vi "Read.vi"(8 "error in (no error)":errorcluster, 9 "timeout (2000 ms)":i32=2000, 10 "bytes to read (100)":i32=100, 11 "TCPConnection in":refnum<class "Connection.lvclass">) -> (0 "error out":errorcluster, 1 "timed out":bool, 2 "Bytes":u8[](array[numeric]) format="%08b", 3 "TCPConnection out":refnum<class "Connection.lvclass">, 4 "connected":bool)   [LabVIEW 2013, in "MQTT_Connection.lvlib" / "Connection.lvclass"]
uses:
  Connection.lvclass
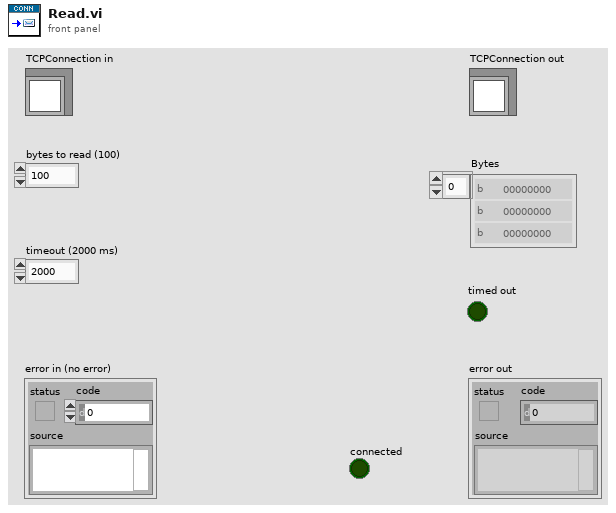
[diagram p1: front panel]
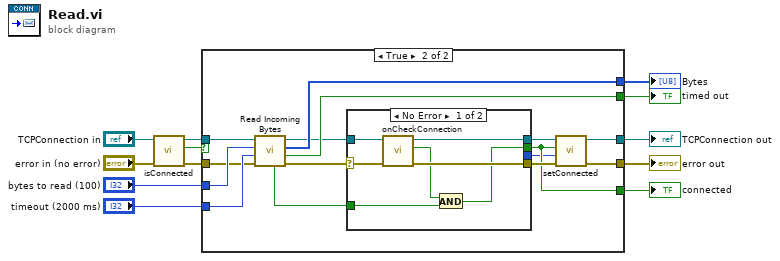
[diagram p0: block diagram]
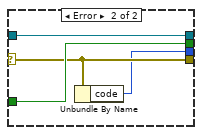
[diagram p3: hidden frame]
diagram:
  n1 = call "isConnected.vi"("error in (no error)"="error in (no error)", "Connection in"="TCPConnection in") -> ("error out"=w2:errorcluster, "connected"=w1:bool, "Connection out"=w4:refnum<class "Connection.lvclass">)  [unwired: 7 in]
  n2 = case shown="True" w1 {
    tunnel: "bytes to read (100)" -> [_ w29]
    tunnel: "timeout (2000 ms)" -> [_ w28]
    tunnel: [_ w27] -> w10
    tunnel: [_ w26] -> w9
    tunnel: [w14 w25] -> w8
    tunnel: [w13 w24] -> w7
    tunnel: [_ w19] -> w6
    tunnel: w4 -> [w14 w18]
    tunnel: w2 -> [w13 w17]
    frame False {
    }
    frame True {
      n3 = call-dynamic "Read Incoming Bytes.vi"("error in (no error)"=w17, "timeout (1000 ms)"=w28, "bytes to read (100)"=w29, "Connection in"=w18) -> ("error out"=w16:errorcluster, "timed out"=w26:bool, "Bytes"=w27:u8[], "Connection out"=w22:refnum<class "Connection.lvclass">, "connected"=w20:bool)  [unwired: 3 in]
      n4 = case shown="No Error" w16 {
        selector: w16 -> [w30 w38]
        tunnel: [w36 w38] -> w23
        tunnel: w22 -> [w35 w40]
        tunnel: [w34 w40] -> w21
        tunnel: w20 -> [w32 w39]
        tunnel: [w31 w39] -> w19
        tunnel: [_ w37] -> w15
        frame No Error {
          n5 = call-dynamic "onCheckConnection.vi"("error in (no error)"=w30, "Connection in"=w35) -> ("error out"=w36:errorcluster, "connection OK"=w33:bool, "Connection out"=w34:refnum<class "Connection.lvclass">)  [unwired: 7 in]
          n6 = And(x=w33, y=w32) -> (x .and. y?=w31:bool)
        }
        frame Error {
          n7 = Unbundle By Name(w38) -> ("code"=w37:i32)
        }
      }
      n8 = call "setConnected.vi"("error in (no error)"=w23, "reason"=w15, "connected"=w19, "Connection in"=w21) -> ("error out"=w24:errorcluster, "Connection out"=w25:refnum<class "Connection.lvclass">)  [unwired: 6 in]
    }
  }
  "error out" <- w7
  "TCPConnection out" <- w8
  "Bytes" <- w10
  "timed out" <- w9
  "connected" <- w6
